vi "Construct.vi"(8 "error in (no error)":errorcluster, 11 "CDebugInfo in":refnum<class "CDebugInfo.lvclass">) -> (0 "error out":errorcluster, 3 "CDebugInfo out":refnum<class "CDebugInfo.lvclass">)   [LabVIEW 2020, in "DependencyInspection.lvlib" / "CDebugInfo.lvclass"]
uses:
  CDebugInfo.lvclass
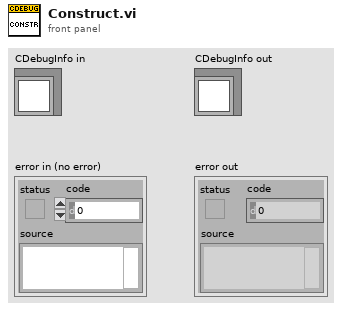
[diagram p1: front panel]
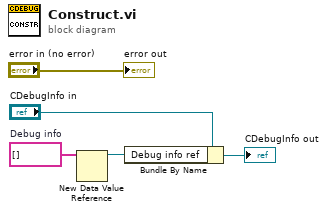
[diagram p0: block diagram]
diagram:
  w4 = string[] []  # Debug info
  n1 = New Data Value Reference(data value=w4) -> (data value reference=w2:refnum<data-value>)  [unwired: 1 in, 1 out]
  n2 = Bundle By Name(cluster="CDebugInfo in", "Debug info ref"=w2) -> (→"CDebugInfo out":refnum<class "CDebugInfo.lvclass">)
  "error out" <- "error in (no error)"
